vi "FFT_polynomial_bkg_standalone.vi"(8 "Y-column names":string[](array[string])=["mr"], 10 "column extension":string[](array[string])=["022", "016"]) -> ()   [LabVIEW 2021]
uses:
  <vilib>/Analysis/1siggen.llb/Ramp Pattern by Samples.vi
  <vilib>/Analysis/4window.llb/Welch Window (DBL).vi
  <vilib>/Analysis/4window.llb/Triangle Window (DBL).vi
  <vilib>/Analysis/4window.llb/Modified Bartlett-Hanning Window (DBL).vi
  <vilib>/Analysis/4window.llb/Hanning Window (DBL).vi
  <vilib>/Analysis/4window.llb/Hamming Window (DBL).vi
  <vilib>/Analysis/4window.llb/Blackman Window (DBL).vi
  <vilib>/Analysis/2dsp.llb/Power Spectrum (DBL).vi
  <vilib>/Analysis/4window.llb/AllCosWindow (DBL).vi
  <vilib>/Analysis/NI_AALPro.lvlib
  <vilib>/Analysis/NI_AALBase.lvlib
  <vilib>/gmath/NI_Gmath.lvlib
panel:
  in  "export":T1(ring)=enum."write to clipboard"
  in  "data offset":dbl format="%.2f"
  in  "use 1/B for fit":bool
  in  "Bbkg final":dbl=2.5 format="%.2f"
  in  "Bbkg init":dbl=1.0 format="%.2f"
  in  "bkg removal method":enum16{"polynomial", "Cheby poly"}(ring)
  out "raw data/bkg":T2(graph)=[{"Ramp Pattern"=[6.58079, 7.15451, 7.7324, 8.21509, 8.81078, 9.28946, 12.64831, 13.13597, 13.63035, 14.11447, 14.6056, 15.0893, 15.57602, 16.06095, 16.54343, 16.91957, 17.40296, 17.87803, 18.35138, 18.81827], "Power Spectrum"=[0.49252, 0.56693, 0.64903, 0.61292, 0.71328, 0.67794, 0.49206, 0.47273, 0.45535, 0.43883, 0.42257, 0.40689, 0.39023, 0.37445, 0.36269, 0.35416, 0.34457, 0.3317, 0.31634, 0.30844]}, {"Ramp Pattern"=[8.21509, 8.81078, 9.28946, 12.64831, 13.13597, 13.63035, 14.11447], "Power Spectrum"=[0.0, 0.0, 0.0, 0.0, 0.0, 0.0, 0.0]}]
  out "FFT spectrum":T2(graph)
  in  "interpol. method":i32(ring)=2 items=["nearest", "linear", "spline", "cubic Hermite", "Lagrange"]
  in  "window":T3(ring)=enum."Hanning"
  in  "stop":bool
  in  "use variables":bool
  in  "Interpolation #":i32=2000
  in  "export spectrum":bool
  out "FFT amp vs variables":string="0.000E+0\t0.000E+0\r\n"
  out "FFTfreq vs variables":string="0.000E+0\t-7.307E-3\r\n"
  out "FFT freq":cluster{"array type (2D Dbl)":dbl[], dbl[]}(graph)={"array type (2D Dbl)"=[0.0], [-0.007307080038623137]}
  out "FFT amp":cluster{"array type (2D Dbl)":dbl[], dbl[]}(graph)
  out "Windowed Signal":cluster{"all rows":dbl[], "all rows":dbl[]}[](graph)=[{"all rows"=[0.125, 0.11904761904761904, 0.1130952380952381, 0.10714285714285714, 0.10119047619047619, 0.09523809523809523, 0.08928571428571427, 0.08333333333333333, 0.07738095238095238, 0.07142857142857142], "all rows"=array[25546 elements]}]
  in  "Bkg poly. order":i32=2
  in  "B final":dbl=14.0 format="%.2f"
  in  "B init":dbl=8.0 format="%.2f"
  out "1/B plot after bkg removed":cluster{"all rows":dbl[], "all rows":dbl[]}[](graph)=[{"all rows"=[0.12172721175300574, 0.11349732940783905, 0.10764888378872399, 0.07906194582517348, 0.07612684864536079, 0.07336568760156563, 0.07084927737279544], "all rows"=[inf, inf, inf, inf, inf, inf, inf]}]
  in  "variable":string="4.2\n3.5\n3"
  # "1. Background removal is done by fitting (normal or Chebyshev polynomial) \n   i) Fitting is done for the range given by 'Bbkg init' and 'Bbkg final'.\n   ii) Background curve is extended to the range give by 'B init' and 'B final'.\n\n2. FFT is done in the range given by 'B init' and 'B final'."
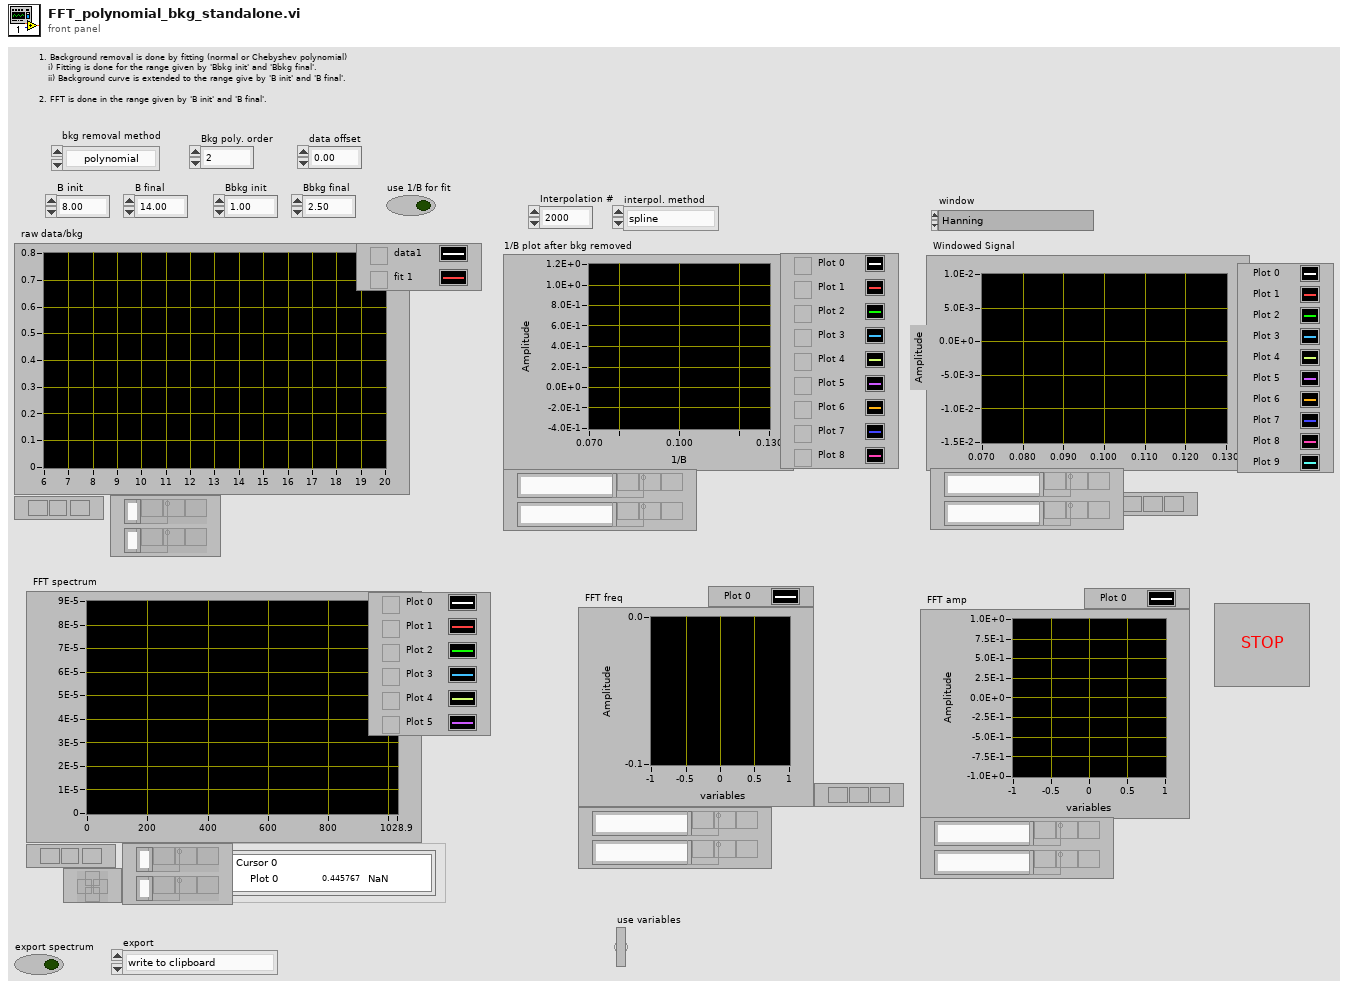
[diagram p1: front panel]
types:
  T1 = enum16{"Save as Ascill file", "write to clipboard", "write to Igor ITX file"}
  T2 = cluster{"Ramp Pattern":dbl[], "Power Spectrum":dbl[]}[]
  T3 = enum16{"none", "Welch", "Triangular", "Bartlett", "Hanning", "Hamming", "Blackmann"}
  T4 = cluster{"array type (2D Dbl)":dbl[], "array type (2D Dbl)":dbl[]}
  T5 = enum16{"Save as Ascill file", "write to clipboard", "do not export"}
  T6 = cluster{"extended B":dbl[], "extended data":dbl[]}
  T7 = cluster{"xi used":dbl[], "Zero Padded Array":dbl[]}
  T8 = cluster{"xi used":dbl[], "Zero Padded Array":dbl[]}[]
  T9 = cluster{"Ramp Pattern":dbl[], "all rows":dbl[]}[]
  T10 = cluster{"extended B":dbl[], "extended data":dbl[]}[]
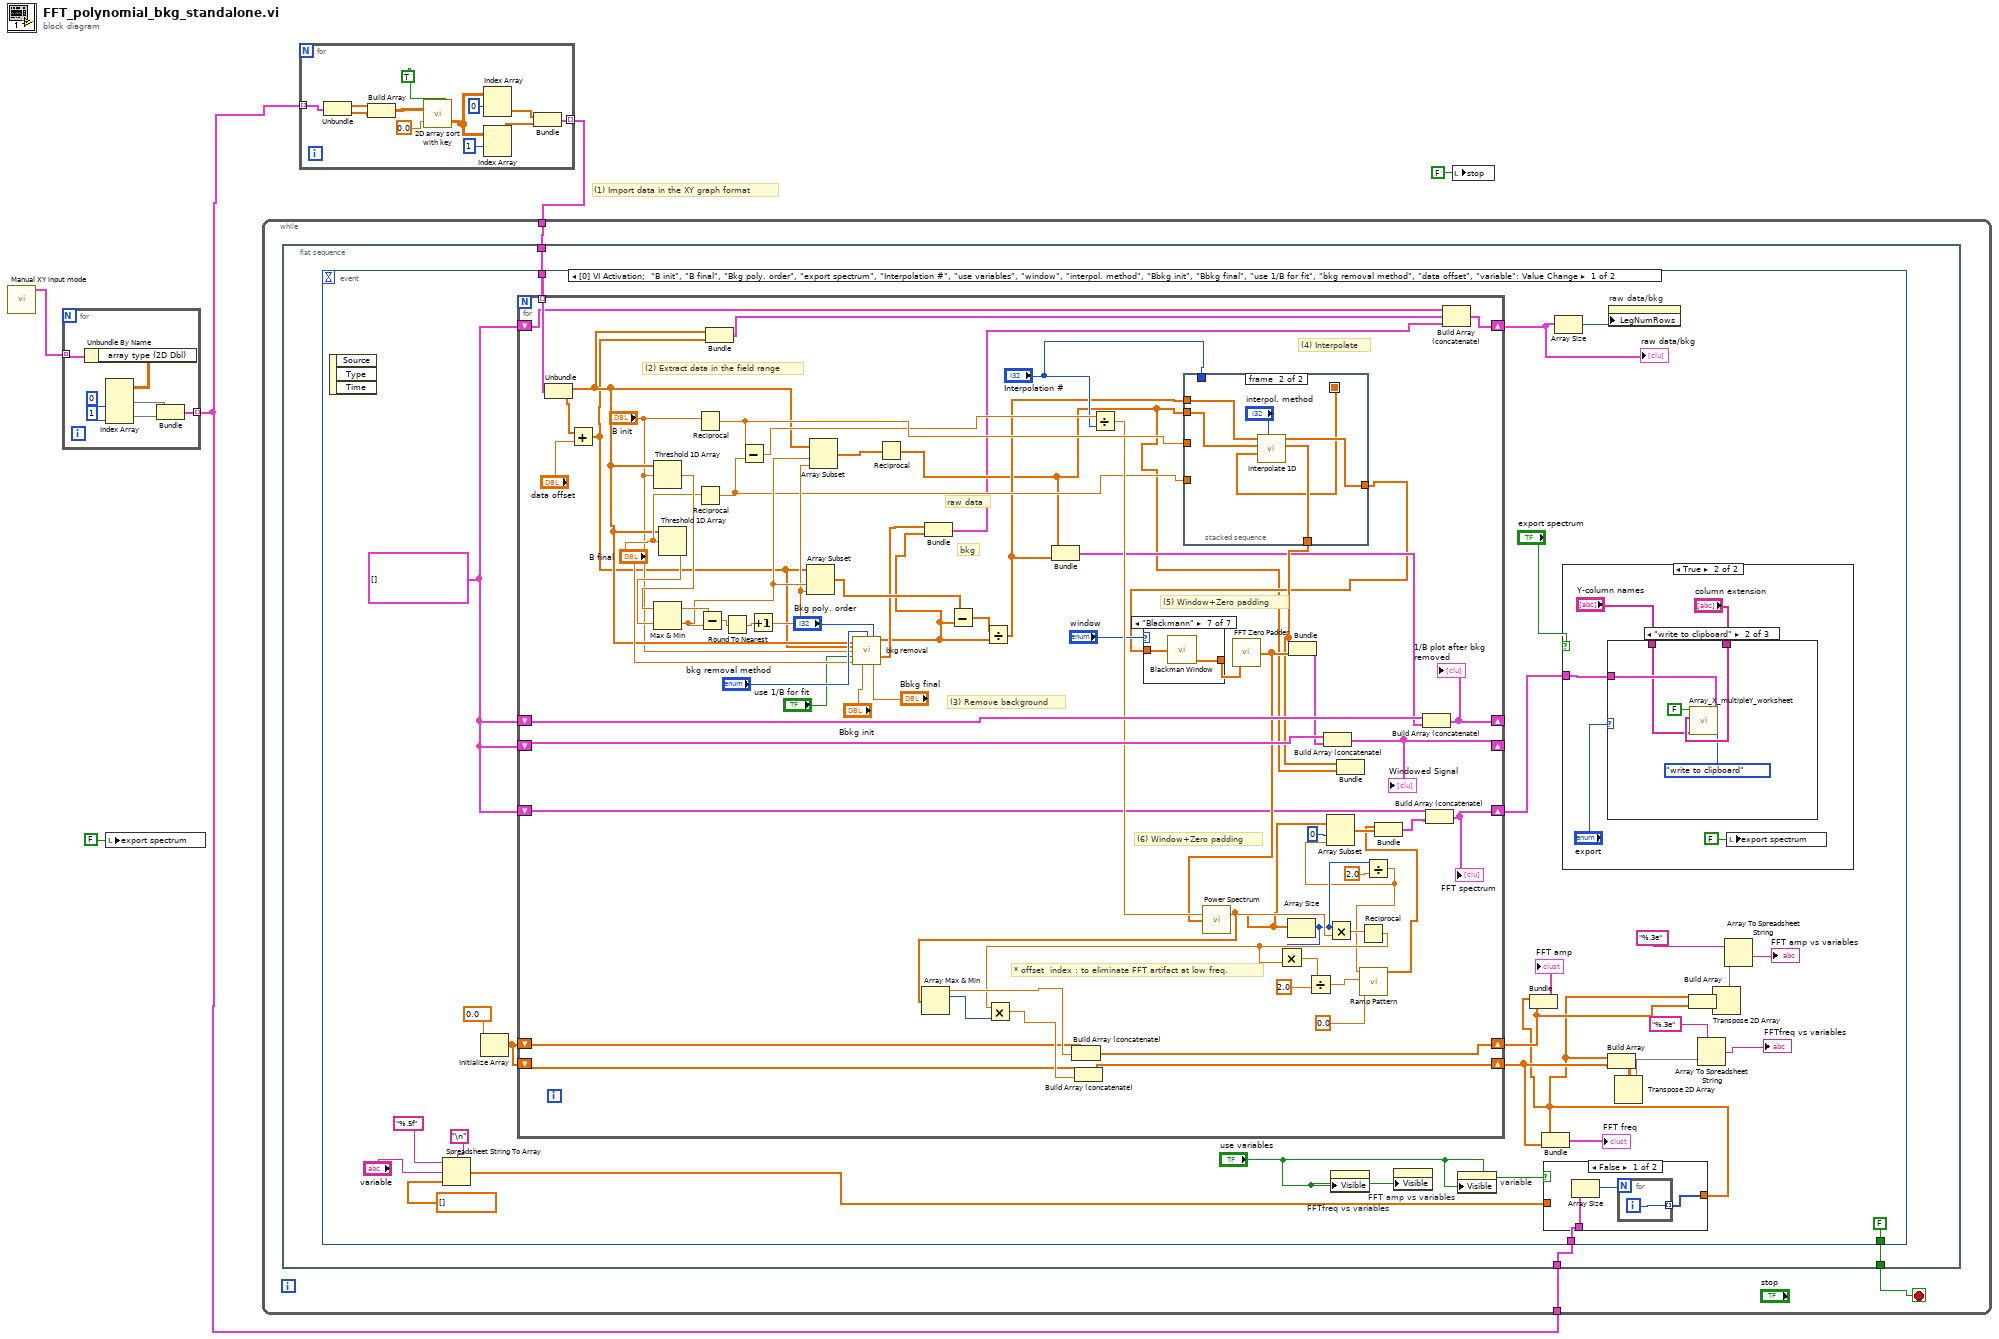
[diagram p0: block diagram]
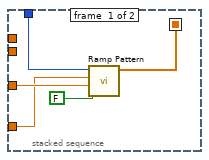
[diagram p3: hidden frame]
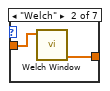
[diagram p5: hidden frame]
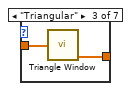
[diagram p6: hidden frame]
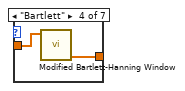
[diagram p7: hidden frame]
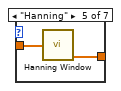
[diagram p8: hidden frame]
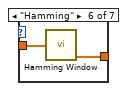
[diagram p9: hidden frame]
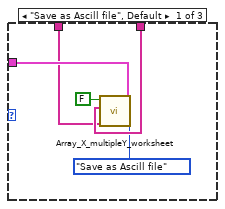
[diagram p11: hidden frame]
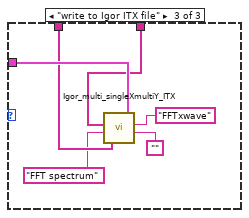
[diagram p12: hidden frame]
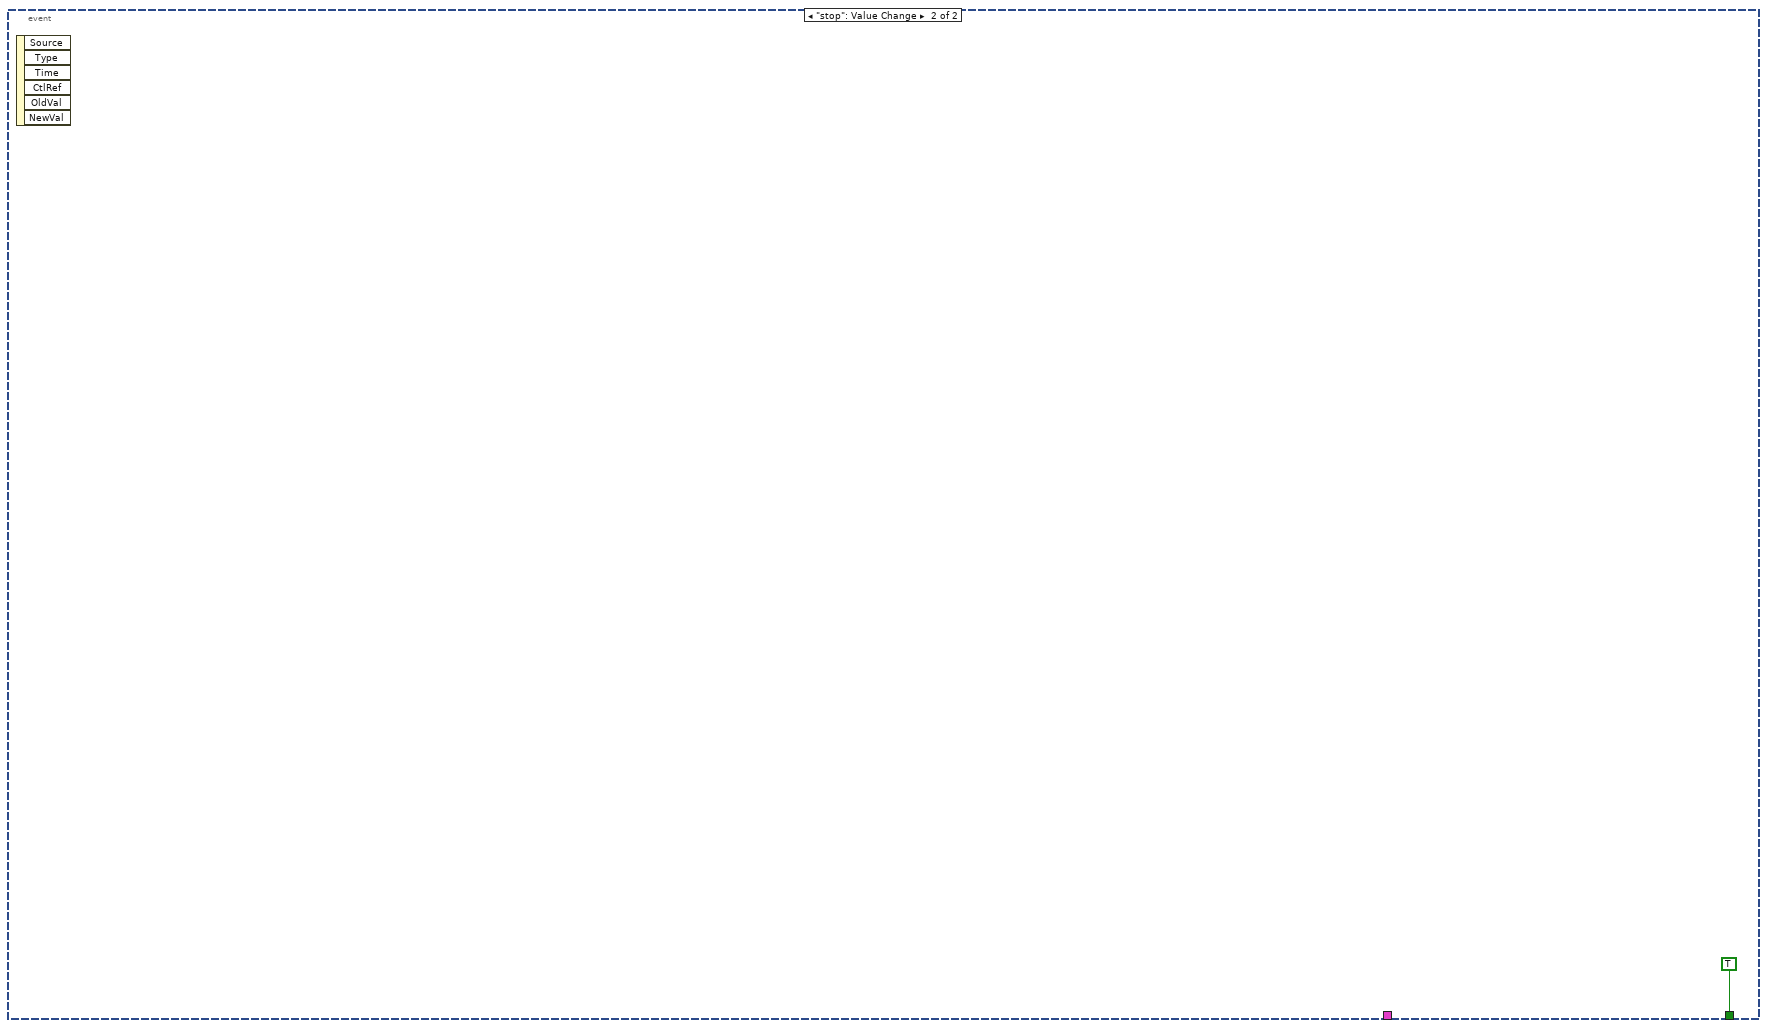
[diagram p13: hidden frame]
diagram:
  # "(1) Import data in the XY graph format"
  n1 = call "Manual XY input mode.vi"() -> ("Data clusters"=w2:cluster{"array type (2D Dbl)":dbl[][]}[])  [unwired: 7 in, 4 out]
  n2 = for {
    tunnel: w2 -> [w12] mode=indexing
    tunnel: [w8] -> w1 mode=indexing
    n3 = Unbundle By Name(w12) -> ("array type (2D Dbl)"=w11:dbl[][])
    n4 = Index Array(array=w11, index (col) #1=0 ("index (row)"), index (col) #2=1 ("index (row)")) -> (element #1=w10:dbl[], element #2=w9:dbl[])  [unwired: 2 in]
    n5 = Bundle("array type (2D Dbl)"=w10, "array type (2D Dbl)"=w9) -> (w8:T4)  [unwired: 1 in]
  }
  n6 = local write "export spectrum"(FALSE ("export spectrum")) -> ()
  n7 = for {
    tunnel: w1 -> [w24] mode=indexing
    tunnel: [w13] -> w4 mode=indexing
    n8 = Unbundle(w24) -> ("array type (2D Dbl)"=w22:dbl[], "array type (2D Dbl)"=w21:dbl[])
    n9 = Build Array(w22, w21) -> (w20:dbl[][])
    n10 = call "2D array sort with key.vi"("ascending"=TRUE, "key row"=0.0, "input"=w20) -> ("output"=w18:dbl[][])
    n11 = Index Array(array=w18, index (row)=0) -> (element=w15:dbl[])  [unwired: 1 in]
    n12 = Index Array(array=w18, index (row)=1) -> (element=w14:dbl[])  [unwired: 1 in]
    n13 = Bundle("output"=w15, "output"=w14) -> (w13:cluster{"output":dbl[], "output":dbl[]})  [unwired: 1 in]
  }
  n14 = while {
    tunnel: w4 -> [w27]
    tunnel: w1 -> [w26]
    stop <- w25 stop-if-true
    n15 = flat-sequence {
      tunnel: w27 -> [w30]
      tunnel: w26 -> [w29]
      tunnel: [w28] -> w25
      frame #0 {
        n16 = event shown="[0] VI Activation;  \"B init\", \"B final\", \"Bkg poly. order\", \"export spectrum\", \"Interpolation #\", \"use variables\", \"window\", \"interpol. method\", \"Bbkg init\", \"Bbkg final\", \"use 1/B for fit\", \"bkg removal method\", \"data offset\", \"variable\": Value Change" {
          selector: _ -> [_ _]
          dyn-events: _ -> [_ _]
          timeout: _ -> [_ _]
          tunnel: w30 -> [w39 _]
          tunnel: w29 -> [w36 _]
          tunnel: [FALSE ("stop (press twice)") TRUE ("stop (press twice)")] -> w28
          event VI Activation; "B init", "B final", "Bkg poly. order", "export spectrum", "Interpolation #", "use variables", "window", "interpol. method", "Bbkg init", "Bbkg final", "use 1/B for fit", "bkg removal method", "data offset", "variable": Value Change {
            w32 = cluster{"all rows":sgl[], "all rows":sgl[]}[] []
            n17 = event-data() -> ()  [unwired: 1 in, 3 out]
            n18 = Spreadsheet String To Array(delimiter (Tab)="\n", format string="%.5f", spreadsheet string="variable", array type (2D Dbl)=dbl[] []) -> (array=w37:dbl[])
            n19 = Initialize Array(0.0 ("element")) -> (w56:dbl[])  [unwired: 1 in]
            n20 = for {
              shift-right: [w114] -> _
              shift-left: w32 -> [w132]
              shift-right: [w113] -> _
              shift-left: w32 -> [w127]
              shift-right: [w89] -> w58
              shift-left: w32 -> [w98]
              shift-right: [w112] -> w48
              shift-left: w56 -> [w116]
              shift-right: [w111] -> w50
              shift-left: w56 -> [w115]
              tunnel: w39 -> [w108] mode=indexing
              shift-right: [w88] -> w35
              shift-left: w32 -> [w87]
              # "(6) Window+Zero padding"
              # "(5) Window+Zero padding"
              # "(4) Interpolate"
              # "(3) Remove background"
              # "(2) Extract data in the field range"
              # "bkg"
              # "raw data"
              # "* offset  index : to eliminate FFT artifact at low freq."
              n21 = Unbundle(w108) -> ("output"=w75:dbl[], "output"=w67:dbl[])
              n22 = Add(x=w67, y="data offset") -> (x+y=w65:dbl[])
              n23 = Threshold 1D Array(2:"B init", 3:w75) -> (0:w131:dbl)  [unwired: 1 in]
              n24 = Threshold 1D Array(2:"B final", 3:w75) -> (0:w130:dbl)  [unwired: 1 in]
              n25 = Max & Min(x=w131, y=w130) -> (max(x,y)=w129:dbl, min(x,y)=w125:dbl)
              n26 = Reciprocal(x="B init") -> (1/x=w124:dbl)
              n27 = Reciprocal(x="B final") -> (1/x=w104:dbl)
              n28 = Subtract(x=w129, y=w125) -> (x-y=w128:dbl)
              n29 = Bundle("output"=w75, w65) -> (w74:cluster{"output":dbl[], dbl[]})  [unwired: 1 in]
              n30 = Round To Nearest(number=w128) -> (nearest integer value=w133:dbl)
              n31 = Subtract(x=w124, y=w104) -> (x-y=w122:dbl)
              n32 = Increment(x=w133) -> (x+1=w123:dbl)
              n33 = Array Subset(array=w65, index=w125, length=w123) -> (w86:dbl[])
              n34 = Array Subset(array=w75, index=w125, length=w123) -> (w73:dbl[])
              n35 = call "bkg removal.vi"("Bfield"=w75, "bkg removal method"="bkg removal method", "poly. order"="Bkg poly. order", "Data"=w65, "B initial"="B init", "inverse"="use 1/B for fit", "B final"="B final", "Bbkg initial"="Bbkg init", "Bbkg final"="Bbkg final") -> ("extended data"=w68:dbl[], "extended B"=w71:dbl[])  [unwired: 4 in, 1 out]
              n36 = Reciprocal(x=w73) -> (1/x=w81:dbl[])
              n37 = Bundle("extended B"=w71, "extended data"=w68) -> (w70:T6)  [unwired: 1 in]
              n38 = Subtract(x=w86, y=w68) -> (x-y=w83:dbl[])
              n39 = Divide(x=w83, y=w68) -> (x/y=w82:dbl[])
              n40 = Bundle(w81, w82) -> (w85:cluster{dbl[], dbl[]})  [unwired: 1 in]
              n41 = Divide(x=w122, y="Interpolation #") -> (x/y=w120:dbl)
              n42 = stacked-sequence {
                seq-local: [w134 _] -> [_ w139]
                tunnel: w82 -> [_ w144]
                tunnel: w81 -> [_ w143]
                tunnel: [_ w142] -> w105
                tunnel: [_ w141] -> w84
                tunnel: "Interpolation #" -> [w138 _]
                tunnel: w124 -> [w137 _]
                tunnel: w104 -> [w136 _]
                frame #0 {
                  n43 = call-poly <vilib>:"Ramp Pattern.vi"("exclude end?"=FALSE, "start"=w137, "end"=w136, "samples"=w138) -> ("Ramp Pattern"=w134:dbl[])  [unwired: 6 in, 1 out]
                }
                frame #1 {
                  n44 = call <vilib>:"Interpolate 1D.vi"("method"="interpol. method", "xi"=w139, "X"=w143, "Y"=w144) -> ("xi used"=w142:dbl[], "yi"=w141:dbl[])  [unwired: 5 in, 1 out]
                }
              }
              n45 = case shown="\"Blackmann\"" "window" {
                tunnel: [w145 w147 w149 w151 w153 w155 w157] -> w121
                tunnel: w84 -> [w145 w146 w148 w150 w152 w154 w156]
                frame "none" {
                }
                frame "Welch" {
                  n46 = call-poly <vilib>:"Welch Window.vi"("X"=w146) -> ("Windowed X"=w147:dbl[])  [unwired: 9 in, 1 out]
                }
                frame "Triangular" {
                  n47 = call-poly <vilib>:"Triangle Window.vi"("X"=w148) -> ("Windowed X"=w149:dbl[])  [unwired: 1 out]
                }
                frame "Bartlett" {
                  n48 = call-poly <vilib>:"Modified Bartlett-Hanning Window.vi"("X"=w150) -> ("Windowed X"=w151:dbl[])  [unwired: 9 in, 1 out]
                }
                frame "Hanning" {
                  n49 = call-poly <vilib>:"Hanning Window.vi"("X"=w152) -> ("Windowed X"=w153:dbl[])  [unwired: 1 out]
                }
                frame "Hamming" {
                  n50 = call-poly <vilib>:"Hamming Window.vi"("X"=w154) -> ("Windowed X"=w155:dbl[])  [unwired: 1 out]
                }
                frame "Blackmann" {
                  n51 = call-poly <vilib>:"Blackman Window.vi"("X"=w156) -> ("Windowed X"=w157:dbl[])  [unwired: 1 out]
                }
              }
              n52 = call "FFT Zero Padder.vi"("Input Array"=w121) -> ("Zero Padded Array"=w119:dbl[])  [unwired: 1 in]
              n53 = call-poly <vilib>:"Power Spectrum.vi"("X"=w119) -> ("Power Spectrum"=w91:dbl[])  [unwired: 1 out]
              n54 = Array Max & Min(array=w91) -> (max value=w118:dbl, max index (indices)=w109:i32)  [unwired: 2 out]
              n55 = Build Array (concatenate)(w116, w118) -> (w112:dbl[])
              n56 = Array Size(array=w91) -> (size(s)=w94:i32)
              n57 = Bundle("xi used"=w105, "Zero Padded Array"=w119) -> (w126:T7)  [unwired: 1 in]
              n58 = Build Array (concatenate)(w127, w126) -> (w113:T8)
              "Windowed Signal" <- w113
              n59 = Multiply(x=w94, y=w120) -> (x*y=w110:dbl)
              n60 = Bundle("xi used"=w105, w81) -> ()  [unwired: 1 in, 1 out]
              n61 = Reciprocal(x=w110) -> (1/x=w103:dbl)
              n62 = Multiply(x=w103, y=w109) -> (x*y=w117:dbl)
              n63 = Build Array (concatenate)(w115, w117) -> (w111:dbl[])
              n64 = Multiply(x=w94, y=w103) -> (x*y=w101:dbl)
              n65 = Divide(x=w101, y=2.0) -> (x/y=w99:dbl)
              n66 = Divide(x=w94, y=2.0) -> (x/y=w90:dbl)
              n67 = Array Subset(array=w91, index=0, length=w90) -> (w93:dbl[])
              n68 = call-poly <vilib>:"Ramp Pattern.vi"("start"=0.0, "end"=w99, "samples"=w90) -> ("Ramp Pattern"=w92:dbl[])  [unwired: 7 in, 1 out]
              n69 = Bundle("Ramp Pattern"=w92, w93) -> (w97:cluster{"Ramp Pattern":dbl[], dbl[]})  [unwired: 1 in]
              n70 = Build Array (concatenate)(w132, w85) -> (w114:cluster{"all rows":dbl[], "all rows":dbl[]}[])
              "1/B plot after bkg removed" <- w114
              n71 = Build Array (concatenate)(w98, w97) -> (w89:T9)
              "FFT spectrum" <- w89
              n72 = Build Array (concatenate)(w87, w74, w70) -> (w88:T10)
            }
            "raw data/bkg" <- w35
            n73 = property on="FFTfreq vs variables" class="Str"("Visible"="use variables") -> ()  [unwired: 2 in, 2 out]
            n74 = property on="FFT amp vs variables" class="Str"("Visible"="use variables") -> ()  [unwired: 2 in, 2 out]
            n75 = property on="variable" class="Str"("Visible"="use variables") -> ()  [unwired: 2 in, 2 out]
            n76 = case shown="False" "use variables" {
              tunnel: w37 -> [_ w64]
              tunnel: [w61 w64] -> w38
              tunnel: w36 -> [w60 _]
              frame False {
                n77 = Array Size(array=w60) -> (size(s)=w62:i32)
                n78 = for {
                  N: w62 -> [_]
                  tunnel: [w63] -> w61 mode=indexing
                  i -> [w63]
                }
              }
              frame True {
              }
            }
            n79 = Bundle("array type (2D Dbl)"=w38, w48) -> (→"FFT amp":cluster{"array type (2D Dbl)":dbl[], dbl[]})  [unwired: 1 in]
            n80 = Bundle("array type (2D Dbl)"=w38, w50) -> (→"FFT freq":cluster{"array type (2D Dbl)":dbl[], dbl[]})  [unwired: 1 in]
            n81 = Array Size(array=w35) -> (size(s)=w34:i32)
            n82 = case shown="True" "export spectrum" {
              tunnel: w58 -> [_ w161]
              frame False {
              }
              frame True {
                n83 = case shown="\"write to clipboard\"" "export" {
                  tunnel: w161 -> [w167 w172 w178]
                  tunnel: "column extension" -> [w165 w170 w177]
                  tunnel: "Y-column names" -> [w164 w169 w176]
                  frame "Save as Ascill file", Default {
                    n84 = call "Array_X_multipleY_worksheet.vi"("export"=T5."Save as Ascill file", "graph file"=w167, "Y-column names"=w164, "column extension"=w165, "Sort?"=FALSE) -> ()  [unwired: 3 in, 2 out]
                  }
                  frame "write to clipboard" {
                    n85 = call "Array_X_multipleY_worksheet.vi"("export"=T5."write to clipboard", "graph file"=w172, "Y-column names"=w169, "column extension"=w170, "Sort?"=FALSE) -> ()  [unwired: 3 in, 2 out]
                  }
                  frame "write to Igor ITX file" {
                    n86 = call "Igor_multi_singleXmultiY_ITX.vi"("message"="", "x-column name"="FFTxwave", "graph file"=w178, "Y-column names"=w176, "window name"="FFT spectrum", "column extension"=w177) -> ()  [unwired: 1 in, 1 out]
                  }
                }
                n87 = local write "export spectrum"(FALSE ("export spectrum")) -> ()
              }
            }
            n88 = Build Array(w38, w50) -> (w55:dbl[][])
            n89 = property on="raw data/bkg" class="XYGraph (strict)"("LegNumRows"=w34) -> ()  [unwired: 2 in, 2 out]
            n90 = Transpose 2D Array(2D array=w55) -> (transposed array=w54:dbl[][])
            n91 = Build Array(w38, w48) -> (w47:dbl[][])
            n92 = Array To Spreadsheet String(array=w54, 3:"%.3e" ("format string")) -> (spreadsheet string=→"FFTfreq vs variables":string)  [unwired: 1 in]
            n93 = Transpose 2D Array(2D array=w47) -> (transposed array=w45:dbl[][])
            n94 = Array To Spreadsheet String(array=w45, 3:"%.3e" ("format string")) -> (spreadsheet string=→"FFT amp vs variables":string)  [unwired: 1 in]
          }
          event "stop": Value Change {
            n95 = event-data() -> ()  [unwired: 1 in, 6 out]
          }
        }
      }
    }
  }
  n96 = local write "stop"(FALSE ("stop")) -> ()
